vi "Apply.vi"(8 "error in (no error)":errorcluster, 11 "DIO DAQmx PWM CFG in":refnum<class "DIO DAQmx PWM CFG.lvclass">) -> (0 "error out":errorcluster, 3 "DIO DAQmx PWM CFG out":refnum<class "DIO DAQmx PWM CFG.lvclass">)   [LabVIEW 2023, in "DAQmx Simulated CFGs.lvlib" / "DIO DAQmx PWM CFG.lvclass"]
uses:
  DIO DAQmx PWM CFG.lvclass
  D:/git/HAL/HAL GOOP4/Configuration JSON Base/CFG JSON Base.lvclass
  Configuration JSON Base/CFG JSON Base.lvclass/CFG JSON Base.ctl
  DIO DAQmx PWM CFG/DIO DAQmx PWM CFG.lvclass
  Configuration JSON Base/CFG JSON Base.lvclass
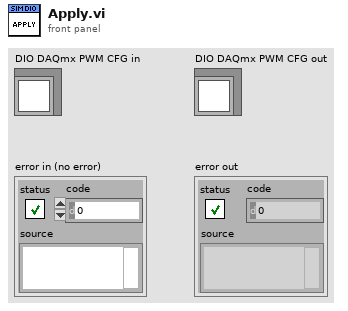
[diagram p1: front panel]
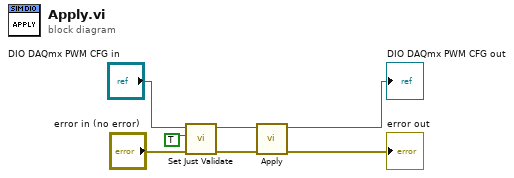
[diagram p0: block diagram]
diagram:
  n1 = call "Set Just Validate.vi"("error in (no error)"="error in (no error)", "Just Validate"=TRUE, "CFG JSON Base in"="DIO DAQmx PWM CFG in") -> ("error out"=w4:errorcluster, "CFG JSON Base out"=w2:refnum<class "DIO DAQmx PWM CFG.lvclass">)  [unwired: 7 in]
  n2 = call-parent "Apply.vi"("error in (no error)"=w4, "DIO DAQmx PWM CFG in"=w2) -> ("error out"=→"error out":errorcluster, "DIO DAQmx PWM CFG out"=→"DIO DAQmx PWM CFG out":refnum<class "DIO DAQmx PWM CFG.lvclass">)  [unwired: 8 in]
